vi "LEDs.vi"(11 "Enum":T1(ring)) -> ()   [LabVIEW 2017]
uses:
  <vilib>/myRIO/Instrument Drivers/Onboard IO/DIO/typedefs/DIO Reference.ctl
  <vilib>/myRIO/Common/Instrument Driver Framework/Utilities/typedefs/myRIO Generic Hardware Reference.ctl
  <vilib>/myRIO/Common/Instrument Driver Framework/Utilities/typedefs/Hardware Version Enum.ctl
  <vilib>/myRIO/Common/Instrument Driver Framework/Utilities/typedefs/myRIO v1.0 Reference.ctl
  <vilib>/myRIO/Common/Instrument Driver Framework/Utilities/typedefs/Generic FPGA Reference.ctl
  <vilib>/myRIO/Common/Instrument Driver Framework/myRIO v1.0/DIO/typedefs/DIO Channels List.ctl
  <vilib>/myRIO/Common/Instrument Driver Framework/myRIO v1.0/DIO/typedefs/DIO Channels Enum.ctl
  <vilib>/userdefined/High Color/nirio_resource_hc.ctl
  <vilib>/myRIO/Common/Instrument Driver Framework/Utilities/vis/Is FPGA Ref Available.vi
  <vilib>/myRIO/Common/Instrument Driver Framework/myRIO v1.0/DIO/vis/myRIO v1.1 Open DIO.vi
  <vilib>/myRIO/Instrument Drivers/Onboard IO/DIO/vis/Write.vi
  <vilib>/myRIO/Common/Instrument Driver Framework/Utilities/vis/Validate Channels.vi
  <vilib>/myRIO/Common/Instrument Driver Framework/myRIO v1.0/DIO/vis/myRIO v1.0 Reserve DIO.vi
  <vilib>/myRIO/Common/Instrument Driver Framework/myRIO v1.0/Resource Manager/vis/myRIO v1.0 Reserve Channel List.vi
  <vilib>/myRIO/Common/Instrument Driver Framework/myRIO v1.0/DIO/vis/myRIO v1.0 Build MUX Configuration DIO.vi
  <vilib>/myRIO/Common/Instrument Driver Framework/myRIO v1.0/Resource Manager/vis/myRIO v1.0 Reserve Channel.vi
  <vilib>/myRIO/Common/Instrument Driver Framework/myRIO v1.0/Resource Manager/vis/myRIO v1.0 Unreserve Channel.vi
  <vilib>/myRIO/Common/Instrument Driver Framework/myRIO v1.0/Resource Manager/vis/myRIO v1.0 Create Configuration List.vi
  <vilib>/myRIO/Common/Instrument Driver Framework/myRIO v1.0/Resource Manager/vis/myRIO v1.0 Build Mutex Name.vi
  <vilib>/Utility/VariantDataType/GetNumericInfo.vi
  <vilib>/Utility/error.llb/Error Cluster From Error Code.vi
  <vilib>/myRIO/Common/Instrument Driver Framework/myRIO v1.0/myRIO v1.1 Open.vi
  <vilib>/myRIO/Common/Instrument Driver Framework/Utilities/vis/IO Manager.vi
  <vilib>/myRIO/Common/Instrument Driver Framework/Utilities/vis/Configuration Manager.vi
  <vilib>/myRIO/Common/Instrument Driver Framework/myRIO v1.0/Resource Manager/vis/myRIO v1.0 Configure IO.vi
  <vilib>/myRIO/Common/Instrument Driver Framework/myRIO v1.0/myRIO v1.0 Close.vi
  <vilib>/myRIO/Common/Instrument Driver Framework/myRIO v1.0/DIO/vis/myRIO v1.0 Write DIO.vi
  <vilib>/myRIO/Express VI/Onboard IO/DO/DO Express VI.xnode
  <vilib>/myRIO/Instrument Drivers/Onboard IO/DIO/vis/myRIO DIO Open.xnode
  <vilib>/myRIO/Instrument Drivers/Onboard IO/DIO/DIO.lvlib
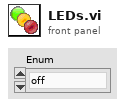
[diagram p1: front panel]
types:
  T1 = enum16{"off", "flash", "top", "middle", "bottom"}
  T2 = typedef "DIO.lvlib/DIO Reference.ctl" = cluster{"myRIO Reference":T3, "DIO Channels List":T7}
  T3 = typedef "myRIO Generic Hardware Reference.ctl" = cluster{"myRIO Model":T4, "myRIO Hardware Reference":T5}
  T4 = typedef "Hardware Version Enum.ctl" = enum16{"Unknown", "myRIO-1900", "myRIO-1950", "roboRIO", "NI ELVIS RIO CM"}
  T5 = typedef "myRIO v1.0 Reference.ctl" = cluster{"Generic FPGA Reference":T6, "Allow multiple opens":bool}
  T6 = typedef "Generic FPGA Reference.ctl" = refnum<k20>
  T7 = typedef "DIO Channels List.ctl" = T8[]
  T8 = typedef "DIO Channels Enum.ctl" = enum16{"Not Connected", "C/DIO0", "C/DIO1", "C/DIO2", "C/DIO3", "C/DIO4", "C/DIO5", "C/DIO6", "C/DIO7", "A/DIO0", "A/DIO1", "A/DIO2", "A/DIO3", "A/DIO4", "A/DIO5", "A/DIO6", "A/DIO7", "A/DIO8", "A/DIO9", "A/DIO10", "A/DIO11", "A/DIO12", "A/DIO13", "A/DIO14", "A/DIO15", "B/DIO0", "B/DIO1", "B/DIO2", "B/DIO3", "B/DIO4", "B/DIO5", "B/DIO6", "B/DIO7", "B/DIO8", "B/DIO9", "B/DIO10", "B/DIO11", "B/DIO12", "B/DIO13", "B/DIO14", "B/DIO15", "LED0", "LED1", "LED2", "LED3", "Button0", "DIO/DIO0", "DIO/DIO1", "DIO/DIO2", "DIO/DIO3", "DIO/DIO4", "DIO/DIO5", "DIO/DIO6", "DIO/DIO7", "DIO/DIO8", "DIO/DIO9", "SPI/CS0", "SPI/CS1", "SPI/CS2", "SPI/CS3", "LED RADIO (Green)", "LED RADIO (Red)", "LED COMM (Green)", "LED COMM (Red)", "LED MODE (Green)", "LED MODE (Red)"}
  T9 = typedef "nirio_resource_hc.ctl" = tag
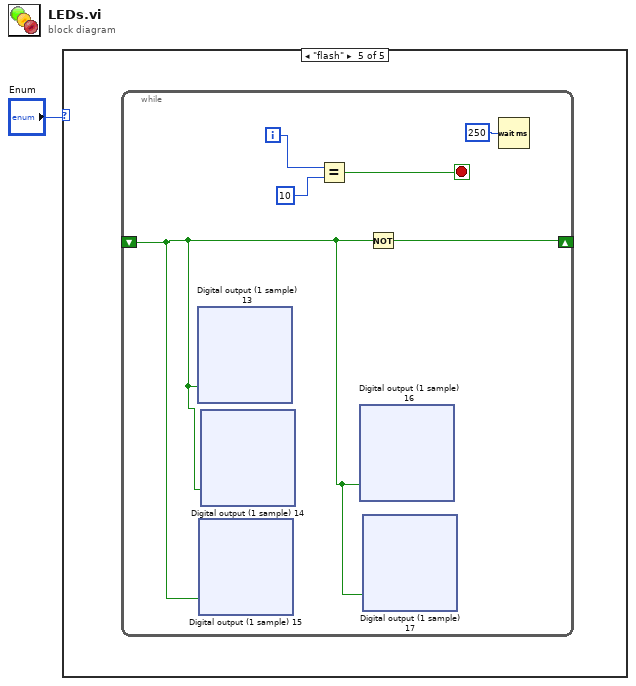
[diagram p0: block diagram]
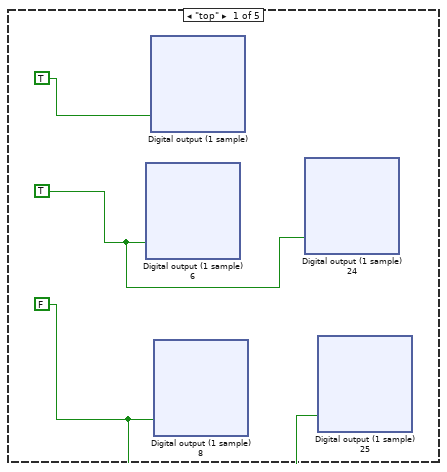
[diagram p2: hidden frame]
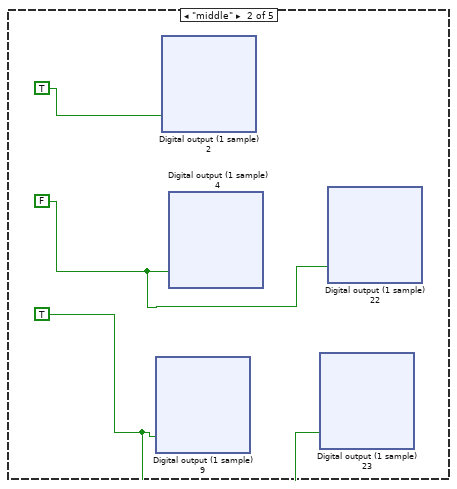
[diagram p3: hidden frame]
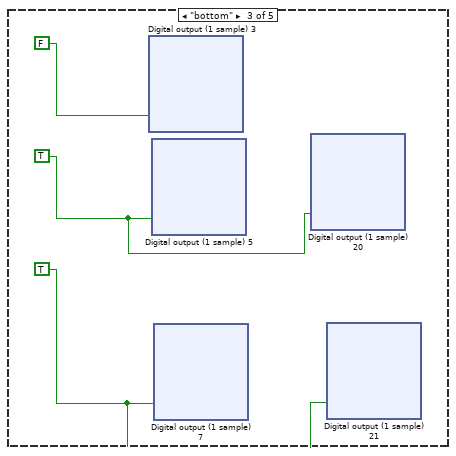
[diagram p4: hidden frame]
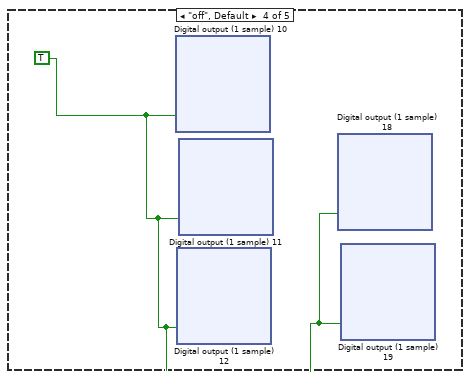
[diagram p5: hidden frame]
diagram:
  n1 = case shown="\"flash\"" "Enum" {
    frame "top" {
      w3 = TRUE ("YELLOW (A/DIO1 (Pin 13))")
      w4 = FALSE ("GREEN (A/DIO0 (Pin 11))")
      n2 = xnode "Digital output (1 sample) 6"("YELLOW (B/DIO7 (Pin 25))"=w3) -> ()  [unwired: 1 in, 1 out]
      n3 = xnode "Digital output (1 sample)"("RED (B/DIO5 (Pin 21))"=TRUE ("RED (A/DIO2 (Pin 15))")) -> ()  [unwired: 1 in, 1 out]
      n4 = xnode "Digital output (1 sample) 8"("GREEN (B/DIO8 (Pin 27))"=w4) -> ()  [unwired: 1 in, 1 out]
      n5 = xnode "Digital output (1 sample) 24"("YELLOW (B/DIO6 (Pin 23))"=w3) -> ()  [unwired: 1 in, 1 out]
      n6 = xnode "Digital output (1 sample) 25"("GREEN (B/DIO9 (Pin 29))"=w4) -> ()  [unwired: 1 in, 1 out]
    }
    frame "middle" {
      w180 = TRUE ("GREEN (A/DIO0 (Pin 11))")
      w181 = FALSE ("YELLOW (A/DIO1 (Pin 13))")
      n7 = xnode "Digital output (1 sample) 9"("GREEN (B/DIO8 (Pin 27))"=w180) -> ()  [unwired: 1 in, 1 out]
      n8 = xnode "Digital output (1 sample) 2"("RED (B/DIO5 (Pin 21))"=TRUE ("RED (A/DIO2 (Pin 15))")) -> ()  [unwired: 1 in, 1 out]
      n9 = xnode "Digital output (1 sample) 4"("YELLOW (B/DIO7 (Pin 25))"=w181) -> ()  [unwired: 1 in, 1 out]
      n10 = xnode "Digital output (1 sample) 23"("GREEN (B/DIO9 (Pin 29))"=w180) -> ()  [unwired: 1 in, 1 out]
      n11 = xnode "Digital output (1 sample) 22"("YELLOW (B/DIO6 (Pin 23))"=w181) -> ()  [unwired: 1 in, 1 out]
    }
    frame "bottom" {
      w358 = TRUE ("GREEN (A/DIO0 (Pin 11))")
      w359 = TRUE ("YELLOW (A/DIO1 (Pin 13))")
      n12 = xnode "Digital output (1 sample) 3"("RED (B/DIO5 (Pin 21))"=FALSE ("RED (A/DIO2 (Pin 15))")) -> ()  [unwired: 1 in, 1 out]
      n13 = xnode "Digital output (1 sample) 5"("YELLOW (B/DIO7 (Pin 25))"=w359) -> ()  [unwired: 1 in, 1 out]
      n14 = xnode "Digital output (1 sample) 7"("GREEN (B/DIO8 (Pin 27))"=w358) -> ()  [unwired: 1 in, 1 out]
      n15 = xnode "Digital output (1 sample) 20"("YELLOW (B/DIO6 (Pin 23))"=w359) -> ()  [unwired: 1 in, 1 out]
      n16 = xnode "Digital output (1 sample) 21"("GREEN (B/DIO9 (Pin 29))"=w358) -> ()  [unwired: 1 in, 1 out]
    }
    frame "off", Default {
      w536 = TRUE ("RED (A/DIO2 (Pin 15))")
      n17 = xnode "Digital output (1 sample) 10"("RED (B/DIO5 (Pin 21))"=w536) -> ()  [unwired: 1 in, 1 out]
      n18 = xnode "Digital output (1 sample) 12"("GREEN (B/DIO8 (Pin 27))"=w536) -> ()  [unwired: 1 in, 1 out]
      n19 = xnode "Digital output (1 sample) 11"("YELLOW (B/DIO7 (Pin 25))"=w536) -> ()  [unwired: 1 in, 1 out]
      n20 = xnode "Digital output (1 sample) 18"("YELLOW (B/DIO6 (Pin 23))"=w536) -> ()  [unwired: 1 in, 1 out]
      n21 = xnode "Digital output (1 sample) 19"("GREEN (B/DIO9 (Pin 29))"=w536) -> ()  [unwired: 1 in, 1 out]
    }
    frame "flash" {
      n22 = while {
        shift-right: [w717] -> _
        shift-left: _ -> [w716]
        i -> [w714]
        stop <- w712 stop-if-true
        n23 = xnode "Digital output (1 sample) 13"("RED (B/DIO5 (Pin 21))"=w716) -> ()  [unwired: 1 in, 1 out]
        n24 = xnode "Digital output (1 sample) 15"("GREEN (B/DIO8 (Pin 27))"=w716) -> ()  [unwired: 1 in, 1 out]
        n25 = xnode "Digital output (1 sample) 14"("YELLOW (B/DIO7 (Pin 25))"=w716) -> ()  [unwired: 1 in, 1 out]
        n26 = Equal?(x=w714, y=10) -> (x = y?=w712:bool)
        n27 = xnode "Digital output (1 sample) 16"("YELLOW (B/DIO6 (Pin 23))"=w716) -> ()  [unwired: 1 in, 1 out]
        n28 = xnode "Digital output (1 sample) 17"("GREEN (B/DIO9 (Pin 29))"=w716) -> ()  [unwired: 1 in, 1 out]
        n29 = Not(x=w716) -> (.not. x?=w717:bool)
        n30 = Wait (ms)(milliseconds to wait=u32 250) -> ()  [unwired: 1 out]
      }
    }
  }
